vi "Write Data - String.vi"(5 "Data Block #":u16, 6 "Start Address":T1, 7 "Memory Area":T2 items=["P Area"=128, "I Area"=129, "O Area"=130, "M Area"=131, "DB Area"=132, "Counter"=40, "Timer"=41], 8 "error in (no error)":errorcluster, 10 "String":string, 11 "S7 in":refnum<class "S7NetCom.lvclass">) -> (0 "error out":errorcluster, 3 "S7 out":refnum<class "S7NetCom.lvclass">)   [LabVIEW 2014, in "S7NetCom.lvclass"]
doc: "Writes raw data to the PLC. \n_____\nCopyright (c) 2019 Hampel Software Engineering (HSE), released under BSD license. More info can be found on https://dokuwiki.hampel-soft.com/code/hse/s7netcom. Original code published by Marc Christenson, Sisu Devices."
uses:
  S7NetCom.lvclass
  Controls/S7_Variable_Type.ctl
  Controls/S7_Memory_Area.ctl
  Controls/S7_Start_Address.ctl
panel:
  # "More info on https://dokuwiki.hampel-soft.com/code/hse/s7netcom\n\nCopyright (c) 2019, HAMPEL SOFTWARE ENGINEERING (HSE)\nOriginal code developed by Marc Christenson, Sisu Devices\nAll rights reserved.\n\nRedistribution and use in source and binary forms, with or without\nmodification, are permitted provided that the following conditions are met:\n\n1. Redistributions of source code must retain the above copyright\n   notice, this list of conditions and the following disclaimer.\n\n2. Redistributions in binary form must reproduce the above copyright\n   notice, this list of conditions and the following disclaimer in the\n   documentation and/or other materials provided with the distribution.\n\n3. All advertising materials mentioning features or use of this software\n   must display the following acknowledgement:\n   This product includes software developed by HAMPEL SOFTWARE ENGINEERING.\n\n4. Neither the name of HAMPEL SOFTWARE ENGINEERING nor the\n   names of its contributors may be used to endorse or promote products\n   derived from this software without specific prior written permission.\n\nTHIS SOFTWARE IS PROVIDED BY HAMPEL SOFTWARE ENGINEERING ''AS IS'' AND ANY\nEXPRESS OR IMPLIED WARRANTIES, INCLUDING, BUT NOT LIMITED TO, THE IMPLIED\nWARRANTIES OF MERCHANTABILITY AND FITNESS FOR A PARTICULAR PURPOSE ARE\nDISCLAIMED. IN NO EVENT SHALL HAMPEL SOFTWARE ENGINEERING BE LIABLE FOR ANY\nDIRECT, INDIRECT, INCIDENTAL, SPECIAL, EXEMPLARY, OR CONSEQUENTIAL DAMAGES\n(INCLUDING, BUT NOT LIMITED TO, PROCUREMENT OF SUBSTITUTE GOODS OR SERVICES;\nLOSS OF USE, DATA, OR PROFITS; OR BUSINESS INTERRUPTION) HOWEVER CAUSED AND\nON ANY THEORY OF LIABILITY, WHETHER IN CONTRACT, STRICT LIABILITY, OR TORT\n(INCLUDING NEGLIGENCE OR OTHERWISE) ARISING IN ANY WAY OUT OF THE USE OF THIS\nSOFTWARE, EVEN IF ADVISED OF THE POSSIBILITY OF SUCH DAMAGE."
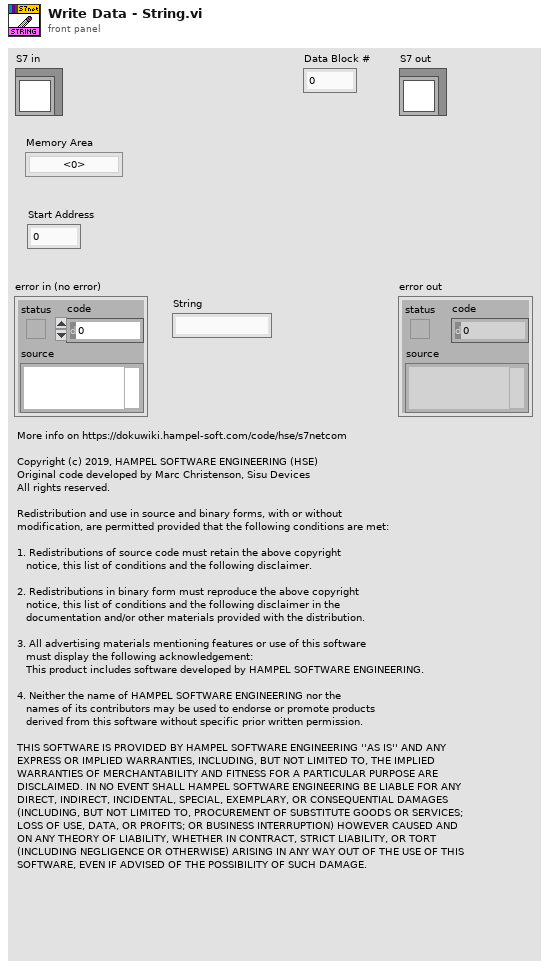
[diagram p1: front panel]
types:
  T1 = typedef "S7NetCom.lvclass/S7_Start_Address.ctl" = u16
  T2 = typedef "S7NetCom.lvclass/S7_Memory_Area.ctl" = u8
  T3 = typedef "S7NetCom.lvclass/S7_Variable_Type.ctl" = enum8{"---", "BIT", "BYTE", "CHAR", "WORD", "INT", "DWORD", "DINT", "REAL"}
  T4 = typedef "S7NetCom.lvclass/S7NetCom_HexByteArray.ctl" = T5[]
  T5 = typedef "S7NetCom.lvclass/S7NetCom_HexByte.ctl" = u8
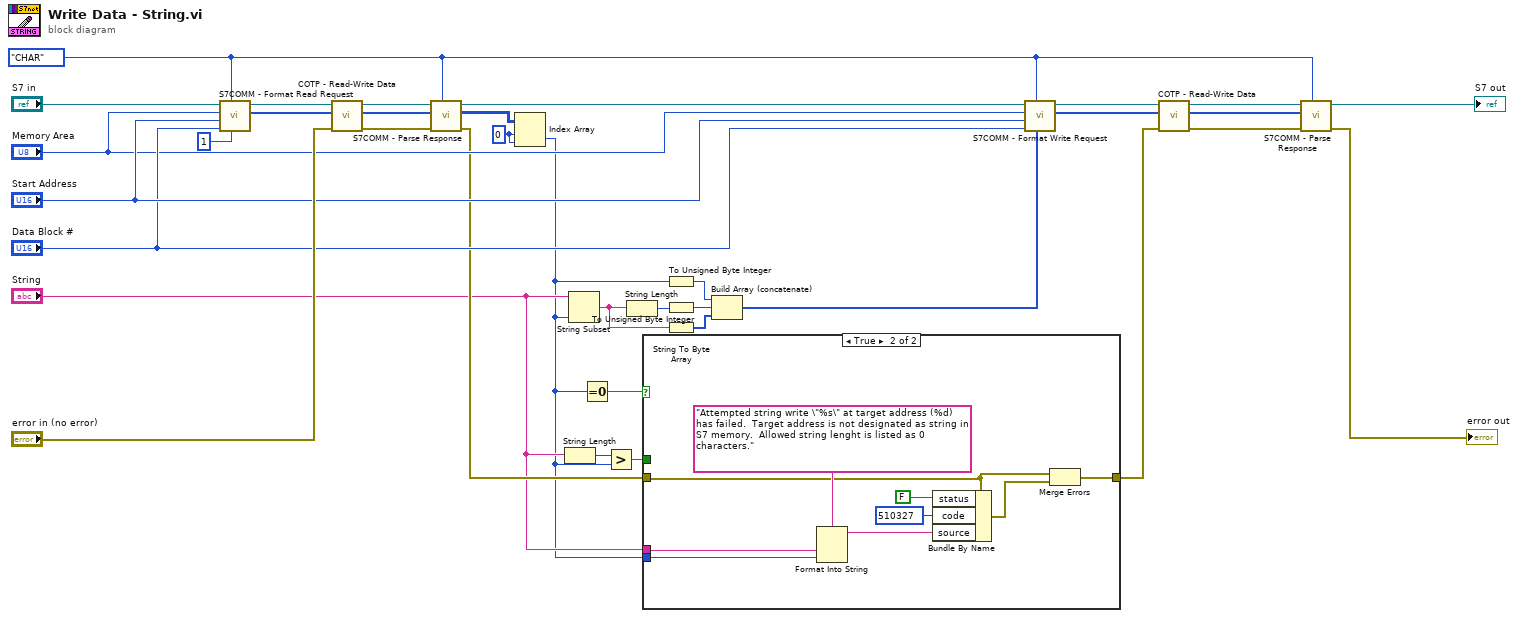
[diagram p0: block diagram]
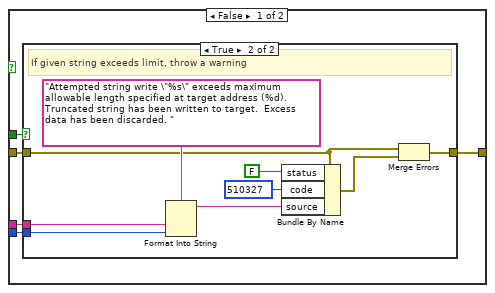
[diagram p2: hidden frame]
diagram:
  w14 = 0 ("index (row)")
  w20 = S7_Variable_Type."CHAR" ("Variable Type")
  n1 = call "S7COMM - Format Read Request.vi"("Read Length"=u16 1, "Variable Type"=w20, "Data Block #"="Data Block #", "Start Address"="Start Address", "Memory Area"="Memory Area", "S7"="S7 in") -> ("S7 PDU Data"=w25:T4, "S7 out"=w26:refnum<class "S7NetCom.lvclass">)  [unwired: 4 in]
  n2 = call "COTP - Read-Write Data.vi"("error in (no error)"="error in (no error)", "S7 PDU in"=w25, "S7 in"=w26) -> ("error out"=w28:errorcluster, "S7 PDU out"=w27:T4, "S7 out"=w24:refnum<class "S7NetCom.lvclass">)  [unwired: 6 in]
  n3 = call "S7COMM - Parse Response.vi"("Variable Type"=w20, "error in (no error)"=w28, "S7 PDU Data"=w27, "S7"=w24) -> ("error out"=w4:errorcluster, "Data Array"=w15:i32[][], "S7 out"=w22:refnum<class "S7NetCom.lvclass">)  [unwired: 4 in, 1 out]
  n4 = Index Array(array=w15, index (row)=w14, index (col)=w14) -> (element=w2:i32)
  n5 = String Length(string="String") -> (length=w6:i32)
  n6 = String Subset(string="String", length (rest)=w2) -> (substring=w9:string)  [unwired: 1 in]
  n7 = Equal To 0?(x=w2) -> (x = 0?=w1:bool)
  n8 = Greater?(x=w6, y=w2) -> (0:w7:bool)
  n9 = String Length(string=w9) -> (length=w10:i32)
  n10 = case shown="True" w1 {
    tunnel: w7 -> [w40 _]
    tunnel: [w39 w53] -> w5
    tunnel: w4 -> [w38 w54]
    tunnel: "String" -> [w37 w52]
    tunnel: w2 -> [w36 w51]
    frame False {
      n11 = case shown="True" w40 {
        tunnel: [w41 w42] -> w39
        tunnel: w38 -> [w41 w49]
        tunnel: w37 -> [_ w45]
        tunnel: w36 -> [_ w44]
        frame False {
        }
        frame True {
          # "If given string exceeds limit, throw a warning"
          n12 = Format Into String(format string="Attempted string write \"%s\" exceeds maximum allowable length specified at target address (%d).  Truncated string has been written to target.  Excess data has been discarded. ", w45, w44) -> (resulting string=w46:string)  [unwired: 2 in, 1 out]
          n13 = Bundle By Name(cluster=w49, "status"=FALSE, "code"=510327, "source"=w46) -> (w43:errorcluster)
          n14 = Merge Errors(w49, w43) -> (w42:errorcluster)
        }
      }
    }
    frame True {
      n15 = Format Into String(format string="Attempted string write \"%s\" at target address (%d) has failed.  Target address is not designated as string in S7 memory.  Allowed string lenght is listed as 0 characters.", w52, w51) -> (resulting string=w59:string)  [unwired: 2 in, 1 out]
      n16 = Bundle By Name(cluster=w54, "status"=FALSE, "code"=510327, "source"=w59) -> (w58:errorcluster)
      n17 = Merge Errors(w54, w58) -> (w53:errorcluster)
    }
  }
  n18 = To Unsigned Byte Integer(number=w2) -> (unsigned 8bit integer=w13:u8)
  n19 = To Unsigned Byte Integer(number=w10) -> (unsigned 8bit integer=w12:u8)
  n20 = String To Byte Array(string=w9) -> (unsigned byte array=w11:u8[])
  n21 = Build Array (concatenate)(w13, w12, w11) -> (w8:u8[])
  n22 = call "S7COMM - Format Write Request.vi"("Data"=w8, "Variable Type"=w20, "Data Block #"="Data Block #", "Start Address"="Start Address", "Memory Area"="Memory Area", "S7"=w22) -> ("S7 PDU Data"=w34:T4, "S7 out"=w32:refnum<class "S7NetCom.lvclass">)  [unwired: 4 in]
  n23 = call "COTP - Read-Write Data.vi"("error in (no error)"=w5, "S7 PDU in"=w34, "S7 in"=w32) -> ("error out"=w30:errorcluster, "S7 PDU out"=w31:T4, "S7 out"=w35:refnum<class "S7NetCom.lvclass">)  [unwired: 6 in]
  n24 = call "S7COMM - Parse Response.vi"("Variable Type"=w20, "error in (no error)"=w30, "S7 PDU Data"=w31, "S7"=w35) -> ("error out"=→"error out":errorcluster, "S7 out"=→"S7 out":refnum<class "S7NetCom.lvclass">)  [unwired: 4 in, 2 out]
